vi "Initialise.vi"(8 "error in (no error)":errorcluster, 11 "Node in":refnum<class "bt_Parallel_Threaded.lvclass">) -> (0 "error out":errorcluster, 3 "Node out":refnum<class "bt_Parallel_Threaded.lvclass">)   [LabVIEW 2021, in "BT.lvlib" / "bt_Parallel_Threaded.lvclass"]
uses:
  bt_Parallel_Threaded.lvclass
  C:/Users/Tim/Documents/GitHub/LV_Behaviour_Tree/Source/Support/Nodes/Composites/abs_Composite/bt_Composite.lvclass
  abs_Composite/bt_Composite.lvclass/bt_Composite.ctl
  System/bt_System.lvclass
  System/bt_System.lvclass/bt_System.ctl
  bt_Parallel_Threaded.lvclass/bt_Parallel_Threaded.ctl
  System/Properties/Write Behaviour Tree.vi
  System/Properties/Write Stop Rendezvous.vi
  abs_Composite/Properties/Read Nodes.vi
  abs_Parallel/bt_Parallel.lvclass
  abs_Node/bt_Node.lvclass
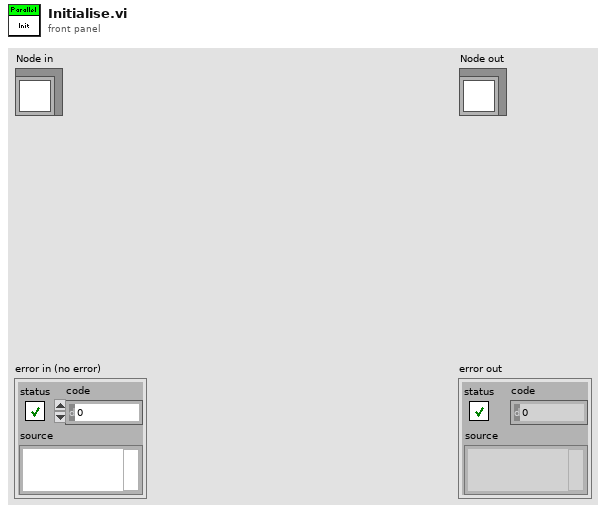
[diagram p1: front panel]
types:
  T1 = typedef "Rendezvous RefNum" = refnum<k1>
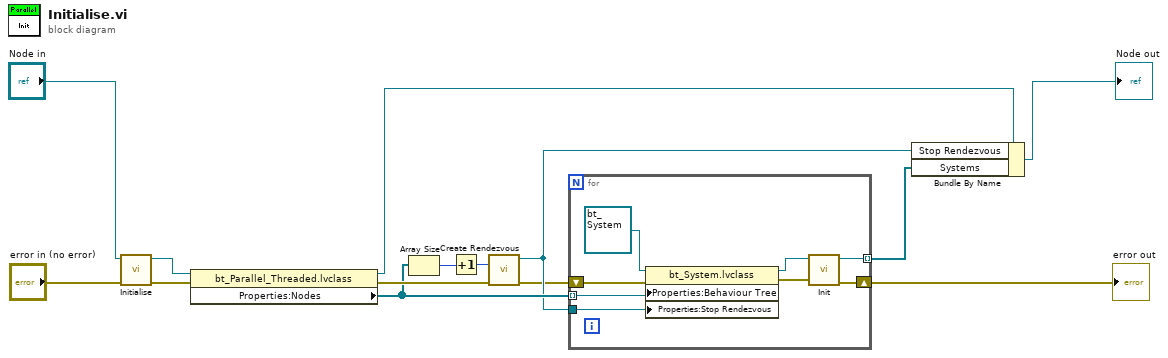
[diagram p0: block diagram]
diagram:
  n1 = call-parent "Initialise.vi"("error in (no error)"="error in (no error)", "Node in"="Node in") -> ("error out"=w12:errorcluster, "Node out"=w11:refnum<class "bt_Parallel_Threaded.lvclass">)  [unwired: 8 in]
  n2 = property class="bt_Parallel_Threaded.lvclass"(reference=w11, error in=w12) -> (reference out=w10:refnum<class "bt_Parallel_Threaded.lvclass">, error out=w6:errorcluster, "Properties:Nodes"=w5:refnum<class "bt_Node.lvclass">[])
  n3 = Array Size(array=w5) -> (size(s)=w3:i32)
  n4 = Increment(x=w3) -> (x+1=w4:i32)
  n5 = call <vilib>:"Create Rendezvous.vi"("error in (no error)"=w6, "size (2)"=w4) -> ("error out"=w1:errorcluster, "rendezvous"=w2:T1)  [unwired: 3 in, 1 out]
  n6 = for {
    shift-right: [w18] -> w8
    shift-left: w1 -> [w22]
    tunnel: w5 -> [w19] mode=indexing
    tunnel: [w17] -> w7 mode=indexing
    tunnel: w2 -> [w16]
    n7 = property class="bt_System.lvclass"(reference=refnum<class "bt_System.lvclass"> refnum ("BT.lvlib:bt_System.lvclass"), error in=w22, "Properties:Behaviour Tree"=w19, "Properties:Stop Rendezvous"=w16) -> (reference out=w20:refnum<class "bt_System.lvclass">, error out=w21:errorcluster)
    n8 = call "Init.vi"("error in (no error)"=w21, "bt_System in"=w20) -> ("error out"=w18:errorcluster, "bt_System out"=w17:refnum<class "bt_System.lvclass">)  [unwired: 8 in]
  }
  "error out" <- w8
  n9 = Bundle By Name(cluster=w10, "Stop Rendezvous"=w2, "Systems"=w7) -> (→"Node out":refnum<class "bt_Parallel_Threaded.lvclass">)
